vi "Audio_Transformation_Setted_Frequency_v001.vi"() -> ()   [LabVIEW 2019]
uses:
  <vilib>/sound2/lvsound2.llb/Sampling Mode.ctl
  <vilib>/sound2/lvsound2.llb/Sound Data Format.ctl
  <vilib>/sound2/lvsound2.llb/Sound Output Set Volume (Single).vi
  <vilib>/addons/Time Frequency Analysis/Transform.llb/TFA Online Gabor Transform (Real).vi
  <vilib>/addons/_Advanced Signal Processing/NI_AdvSigProcTFA.lvlib
panel:
  out "u(t)":dbl(graph)
  out "V(t)":dbl(graph)
  in  "Neuron Type":T1(ring)
  out "max index(es)":i32
  out "max value":dbl
  out "Waveform Graph":dbl[](graph)
  out "Magnitude of Gabor Coefficients":dbl[][](graph)
  in  "Device ID":u32
  in  "Stop":bool
  in  "Frequency":dbl=500.0
  out "Generated Sound":waveform(dbl)(graph)
  in  "Volume":dbl(slide)=50.0 scale=0.0..100.0
  # "Step one: Sound generated by the computer"
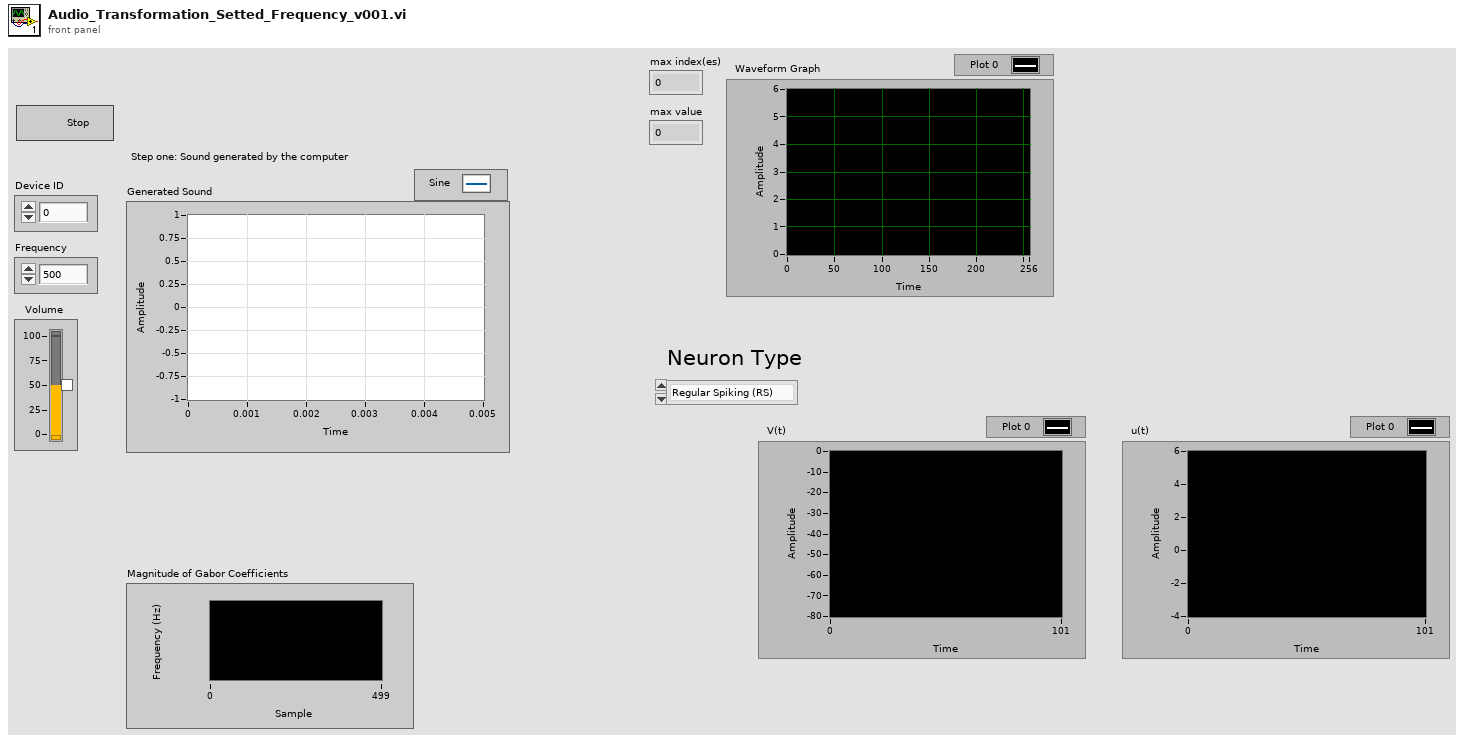
[diagram p1: front panel]
types:
  T1 = enum16{"Regular Spiking (RS)", "Intrinsically Bursting (IB)", "Chattering (CH)", "Fast Spiking (FS)", "Thalamo-Cortical 1 (TC1)", "Thalamo-Cortical 2 (TC2)", "Resonator (RZ)", "Low-Threshold Spiking (LTS)"}
  T2 = typedef "Sound Data Format.ctl" = cluster{"sample rate (S/s)":dbl, "number of channels":i32, "bits per sample":i32}
  T3 = typedef "Sampling Mode.ctl" = i32
  T4 = typedef "Sound Output Task ID.ctl" = u32
  T5 = cluster{"analysis window":dbl[], "dM (time steps)":i32, "N (frequency bins)":i32}
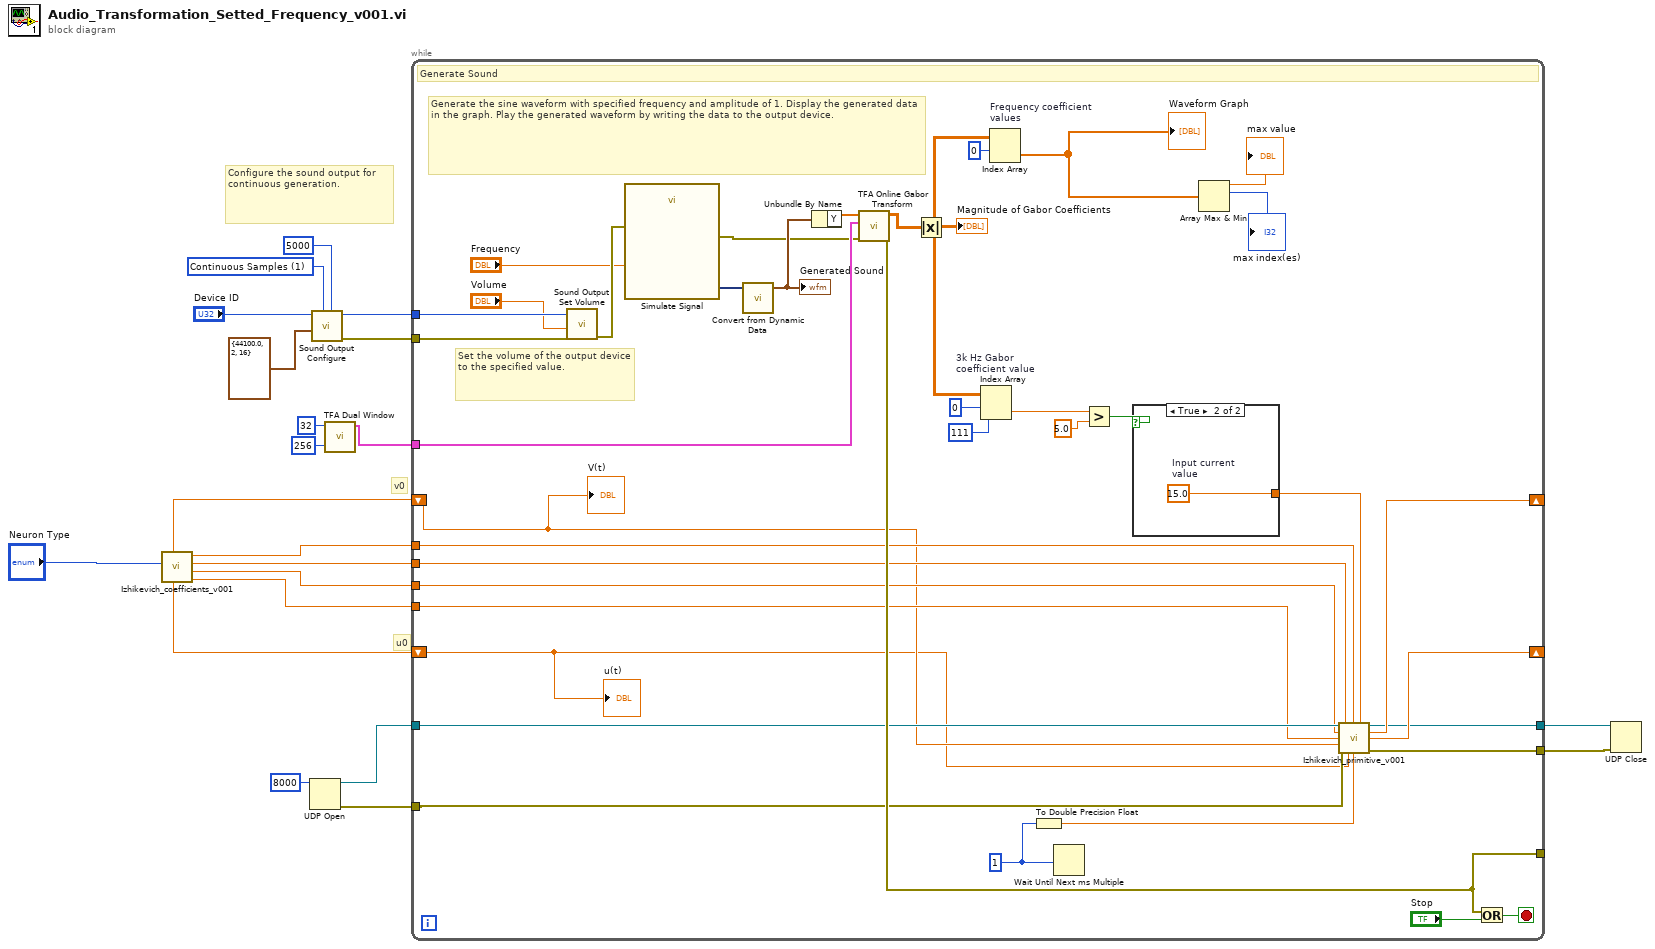
[diagram p0: block diagram]
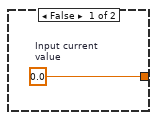
[diagram p2: hidden frame]
diagram:
  w18 = T3 1 items=["Finite Samples", "Continuous Samples"] ("sample mode")
  # "u0"
  # "v0"
  # "Configure the sound output for continuous generation."
  n1 = call "Izhikevich_coefficients_v001.vi"("Neuron Type"="Neuron Type") -> ("d"=w6:dbl, "c"=w7:dbl, "b"=w8:dbl, "a"=w9:dbl, "u0"=w10:dbl, "v0"=w11:dbl)  [unwired: 3 in]
  n2 = UDP Open(11:u16 8000 ("port")) -> (port=w4:refnum<k16>, 0:w3:errorcluster)  [unwired: 4 in, 1 out]
  n3 = call <vilib>:"Sound Output Configure.vi"("number of samples/ch"=5000 ("Number of Samples/ch"), "sample mode"=w18, "sound format"=T2 {"sample rate (S/s)"=44100.0, "number of channels"=2, "bits per sample"=16} ("Sound Format"), "device ID"="Device ID") -> ("error out"=w21:errorcluster, "task ID"=w20:T4)  [unwired: 6 in]
  n4 = call <vilib>:"TFA Dual Window.vi"("N (frequency bins)"=256, "dM (time steps)"=32) -> ("analysis info"=w13:T5)  [unwired: 7 in, 2 out]
  n5 = while {
    tunnel: w20 -> [w57]
    tunnel: w21 -> [w58]
    tunnel: [w40] -> _
    tunnel: w13 -> [w52]
    shift-right: [w27] -> _
    shift-left: w11 -> [w23]
    shift-right: [w26] -> _
    shift-left: w10 -> [w22]
    tunnel: w9 -> [w35]
    tunnel: w8 -> [w34]
    tunnel: w7 -> [w32]
    tunnel: w6 -> [w31]
    tunnel: w4 -> [w33]
    tunnel: w3 -> [w30]
    tunnel: [w25] -> w2
    tunnel: [w24] -> w1
    stop <- w59 stop-if-true
    w29 = u32 1 ("millisecond multiple")
    # "Set the volume of the output device to the specified value."
    # "Generate the sine waveform with specified frequency and amplitude of 1. Display the generated data in the graph. Play the generated waveform by writing the data to the output device."
    # "Generate Sound"
    n6 = call-poly <vilib>:"Sound Output Set Volume.vi"("error in (no error)"=w58, "volume"="Volume", "task ID"=w57) -> ("error out"=w55:errorcluster)  [unwired: 7 in, 1 out]
    n7 = call "Simulate Signal"("Frequency"="Frequency", "error in (no error)"=w55) -> ("Sine"=w54:dynamicdata, "error out"=w48:errorcluster)  [unwired: 12 in]
    n8 = call "Convert from Dynamic Data"("Dynamic Data Type"=w54) -> ("Waveform"=w51:waveform(dbl))  [unwired: 3 in]
    "Generated Sound" <- w51
    n9 = Unbundle By Name(w51) -> ("Y"=w50:dbl[])
    n10 = call-poly <vilib>:"TFA Online Gabor Transform.vi"("error in (no error)"=w48, "transform info"=w52, "signal"=w50) -> ("error out"=w40:errorcluster, "Gabor coef"=w49:cdb[][])  [unwired: 6 in, 1 out]
    n11 = Absolute Value(x=w49) -> (abs(x)=w43:dbl[][])
    "Magnitude of Gabor Coefficients" <- w43
    n12 = Index Array "3k Hz Gabor \ncoefficient value"(array=w43, index (row)=0, index (col)=111 ("disabled index (col)")) -> (element=w39:dbl)
    n13 = Index Array "Frequency coefficient \nvalues"(array=w43, index (row)=0) -> (element=w45:dbl[])  [unwired: 1 in]
    "Waveform Graph" <- w45
    n14 = To Double Precision Float(number=w29) -> (double precision float=w28:dbl)
    n15 = Wait Until Next ms Multiple(millisecond multiple=w29) -> ()  [unwired: 1 out]
    n16 = Greater?(x=w39, y=5.0) -> (0:w37:bool)
    n17 = case shown="True" w37 {
      tunnel: [w61 w62] -> w36
      frame False {
        w61 = 0.0  # Input current  value
      }
      frame True {
        w62 = 15.0  # Input current  value
      }
    }
    n18 = Array Max & Min(array=w45) -> (max value=→"max value":dbl, max index (indices)=→"max index(es)":i32)  [unwired: 2 out]
    n19 = call "Izhikevich_primitive_v001.vi"("UDP Network Connection in"=w33, "b"=w34, "a"=w35, "I"=w36, "c"=w32, "d"=w31, "v(t)"=w23, "error in (no error)"=w30, "u(t)"=w22, "dt"=w28) -> ("UDP Network Connection out"=w24:refnum<k16>, "v(t+dt)"=w27:dbl, "u(t+dt)"=w26:dbl, "error out"=w25:errorcluster)  [unwired: 2 in]
    n20 = Or(x=w40, y="Stop") -> (x .or. y?=w59:bool)
    "V(t)" <- w23
    "u(t)" <- w22
  }
  n21 = UDP Close(connection ID=w1, 8:w2) -> ()  [unwired: 2 out]
